vi "Server_v2.vi"() -> ()   [LabVIEW 2016]
uses:
  <vilib>/rvi/eio/common/nirviEmuClasses.ctl
  <vilib>/rvi/Emulation/niFpgaSctlEmulationGetInTimedLoop.vi
  <vilib>/rvi/Emulation/niFpgaProcessEmulError.vi
  <vilib>/rvi/eio/common/nirviEmuTemplateMethod_errors.vi
  <vilib>/rvi/Emulation/niFpgaEmulationIsFPGAContextNoSignature.vi
  <vilib>/rvi/DataTransferAndStorage/Container/Common/niFpgaContainerGetUniqueNameForEmu.vi
  <vilib>/rvi/Memory/Memory_Emulation/niFpgaMemoryEmulationCacheClearOnFirstRun.vi
  <vilib>/rvi/Memory/Memory_Emulation/nirvimemoryEmulationManagerCache_MakeExclusive.vi
  <vilib>/rvi/Memory/Memory_Emulation/niFpgaMemoryEmulationValidateCache.vi
  <vilib>/rvi/Memory/Memory_Emulation/nirvimemoryEmulationManagerCache_InsertValue.vi
  <vilib>/Utility/error.llb/Clear Errors.vi
  <vilib>/rvi/Memory/Memory_Emulation/nirvimemoryEmulationManagerCache_ReleaseExclusive.vi
  <vilib>/rvi/Memory/Memory_Emulation/nirvimemoryEmulationManagerCache_GetValue.vi
  <vilib>/rvi/Memory/Memory_Emulation/nirvimemoryEmulationManagerCache_SetValue.vi
  <vilib>/rvi/Emulation/niFpgaGetClockAttributes.vi
  <vilib>/rvi/Emulation/niFpgaEmulationReportErrorSimple.vi
  <vilib>/rvi/Emulation/niFpgaCriticalErrorInLSC.vi
  <vilib>/rvi/eio/common/nirviEmuTemplateMethod_noerrors.vi
  <vilib>/rvi/errors/niFpgaSetErrorForExecOnDevCompSimple.vi
  <vilib>/rvi/eio/common/nirviEmuReportErrorAndStop.vi
  <vilib>/rvi/FIFO/Fifo_Resource/nirvififoEmulationSetSize.vi
  <vilib>/rvi/FIFO/Fifo_Resource/nirviFifoEmulationQueueMgr.vi
  <instcachedir>/0/nirviFifoEmulationQueueMgr_E5CAEC123FF24DC58D834DCA3CDAA9B5.lvgen/nirviFifoEmulationQueueMgr_E5CAEC123FF24DC58D834DCA3CDAA9B5_001.vi
  <vilib>/rvi/FIFO/Fifo_Resource/nirvififoEmulationCreateLock.vi
  <vilib>/rvi/FIFO/Fifo_Resource/nirvififoEmulationObtainLock.vi
  <vilib>/rvi/FIFO/Fifo_Resource/nirvififoEmulationReleaseLock.vi
  <vilib>/rvi/occurrence/nirviWaitOnOccurrenceBase.vi
  <vilib>/rvi/errors/nirviReportUnexpectedCaseInternalError.vi
  <vilib>/rvi/errors/nirviReportUnexpectedCaseInternalError (U32).vi
  <vilib>/rvi/FIFO/Fifo_Resource/nirvififoEmulationDetermineInputValidOut.vi
  <vilib>/eio/EIOGrowableMethodNode/genericMethod/EIOGrowableMethodNode.xnode
  <vilib>/rvi/eio/nirviEIOMethodImplementation/nirviEIOMethodImplementation.xnode
  <vilib>/rvi/eio/nirviErrorMerge/nirviErrorMerge.xnode
  <vilib>/rvi/DataTransferAndStorage/Container/XNode/niFpgaContainer.xnode
  <vilib>/rvi/DataTransferAndStorage/Register/Emulation/niFpgaRegisterEmulation.vi
  <vilib>/eio/EIONode/EIONode.xnode
  <vilib>/rvi/FIFO/Fifo_Resource/nirvififoEmulationRead.vi
  <vilib>/rvi/FIFO/Fifo_Resource/nirvififoEmulationWrite.vi
panel:
  out "Temperatures":T1
  in  "Spare DC Relay 1":bool
  in  "AC Spare":bool
  in  "Spare DC Relay 2":bool
  out "Sensor Status":u8
  in  "PAS Laser 1 Enable":bool
  in  "PAS Laser 2 Enable":bool
  in  "CRD Laser Enable":bool
  in  "Fan Voltage":i16
  in  "CRD Heater Enable":bool
  in  "PAS Heater 2":bool
  in  "PAS Heater 1":bool
  in  "pas_frequency":u64
  in  "Vacuum Pump":bool
  in  "Error Mode":bool
  in  "PAS Speaker Enable":bool
  in  "O2 Add":bool
  in  "uv light enable":bool
  in  "Fan Enable":bool
  in  "O3 Add":bool
  in  "Filter Ctl":bool
  in  "Transmit?":bool
  in  "CRDSampData":u32
  in  "Speaker":cluster{"Vscale":fxp<+,32,0>, "Offset":i16}
  in  "Stop":bool
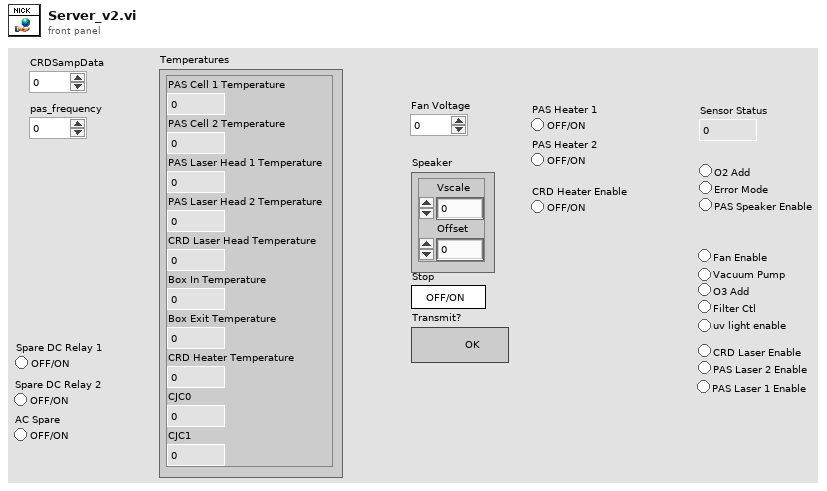
[diagram p1: front panel]
types:
  T1 = cluster{"PAS Cell 1 Temperature":fxp<+/-,24,-2>, "PAS Cell 2 Temperature":fxp<+/-,24,-2>, "PAS Laser Head 1 Temperature":fxp<+/-,24,-2>, "PAS Laser Head 2 Temperature":fxp<+/-,24,-2>, "CRD Laser Head Temperature":fxp<+/-,24,-2>, "Box In Temperature":fxp<+/-,24,-2>, "Box Exit Temperature":fxp<+/-,24,-2>, "CRD Heater Temperature":fxp<+/-,24,-2>, "CJC0":fxp<+/-,24,-2>, "CJC1":fxp<+/-,24,-2>}
  T2 = typedef "nirviEmuClasses.ctl" = enum16{"IO Read", "IO Write", "Method", "Property Read", "Property Write"}
  T3 = cluster{"PAS Cell 1 Temperature":fxp<+/-,24,-2>, "PAS Cell 2 Temperature":fxp<+/-,24,-2>, "PAS Laser Head 1 Temperature":fxp<+/-,24,-2>, "PAS Laser Head 2 Temperature":fxp<+/-,24,-2>, "CRD Laser Head Temperature":fxp<+/-,24,-2>, "Box In Temperature":fxp<+/-,24,-2>, "Box Exit Temperature":fxp<+/-,24,-2>, "CRD Heater Temperature":fxp<+/-,24,-2>, "Mod5/CJC0":fxp<+/-,24,-2>, "Mod5/CJC1":fxp<+/-,24,-2>}
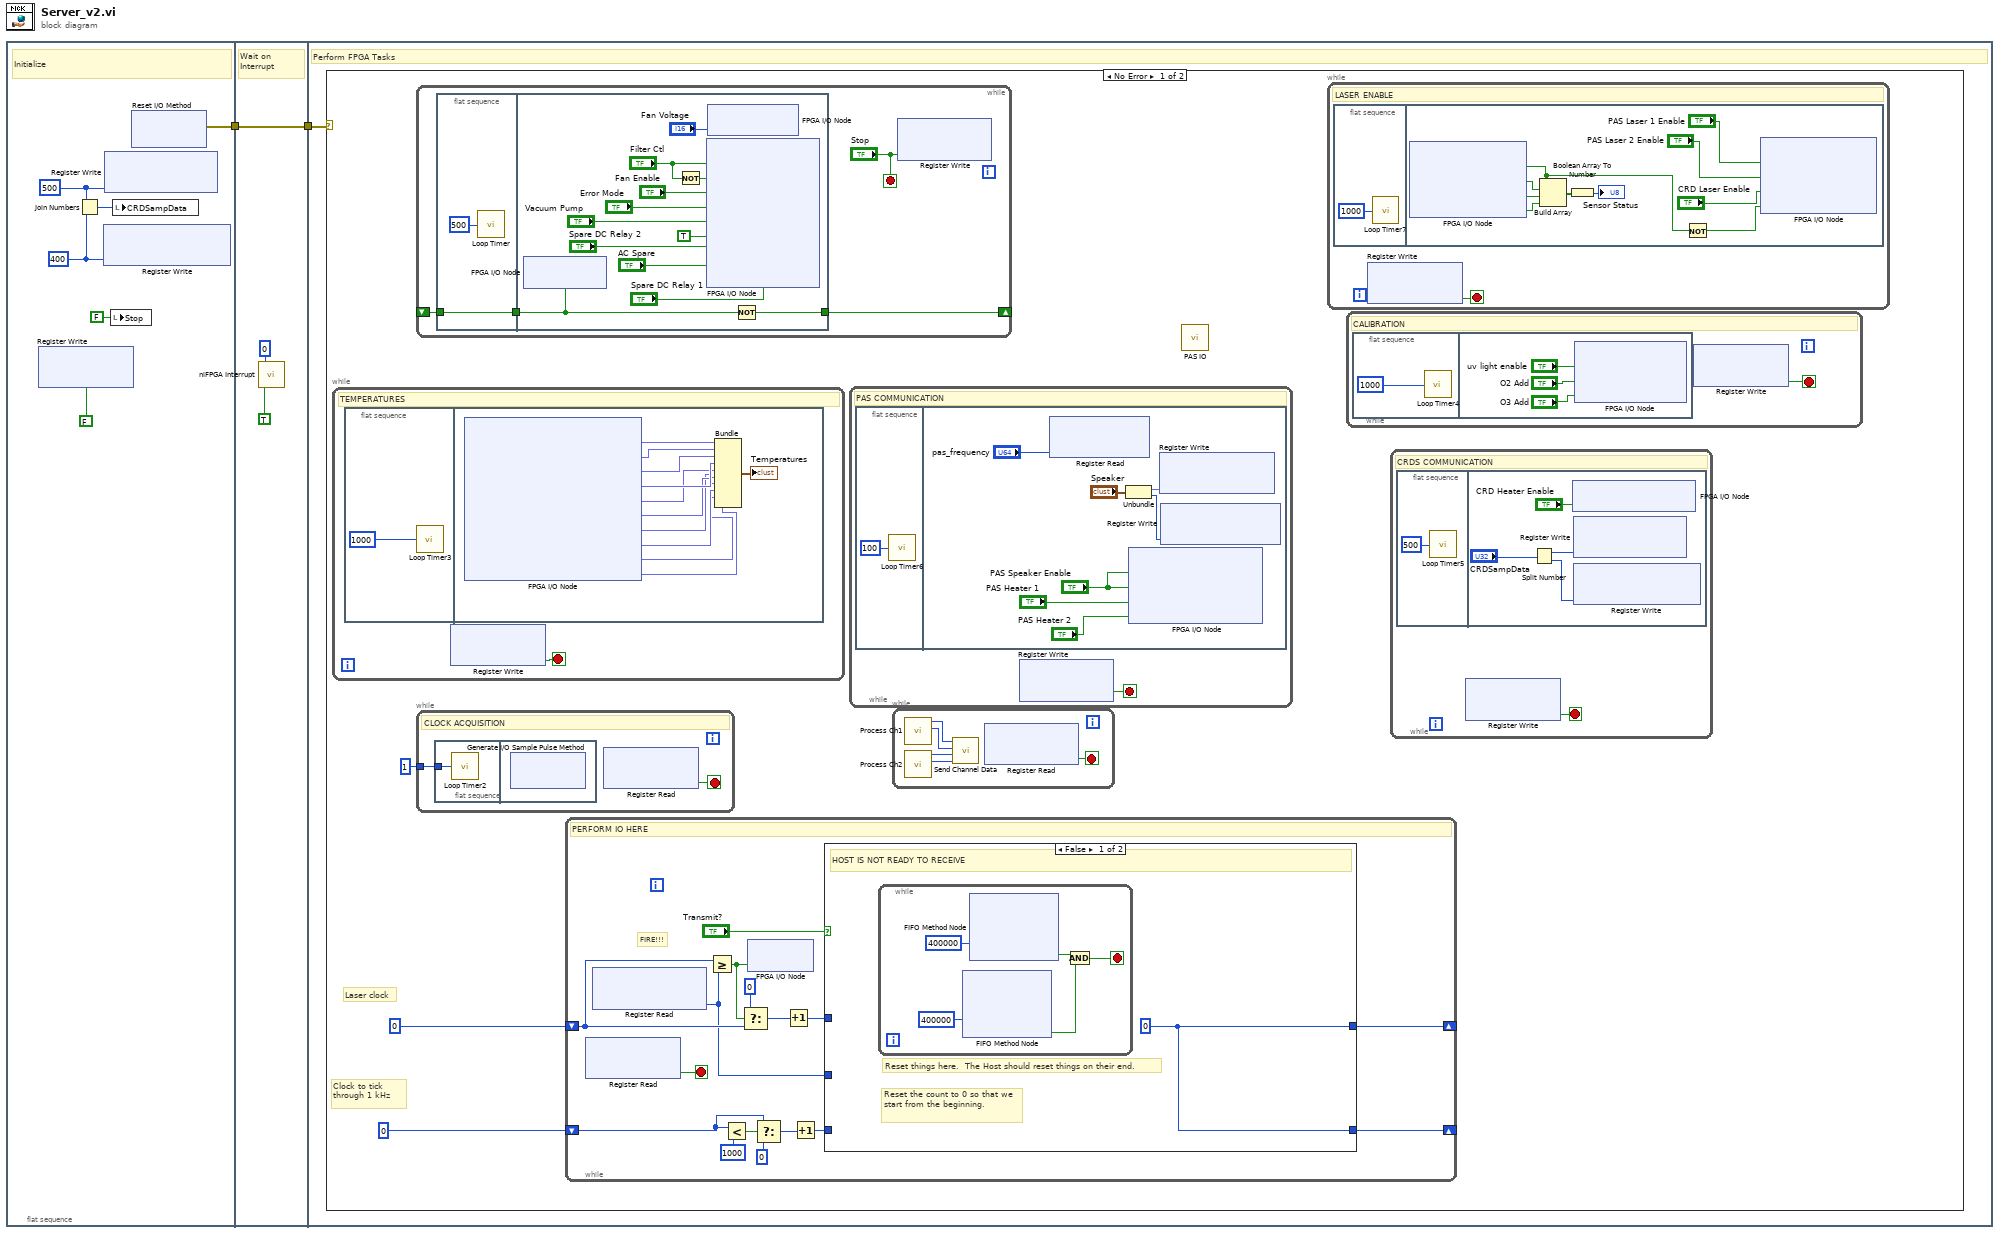
[diagram p0: block diagram]
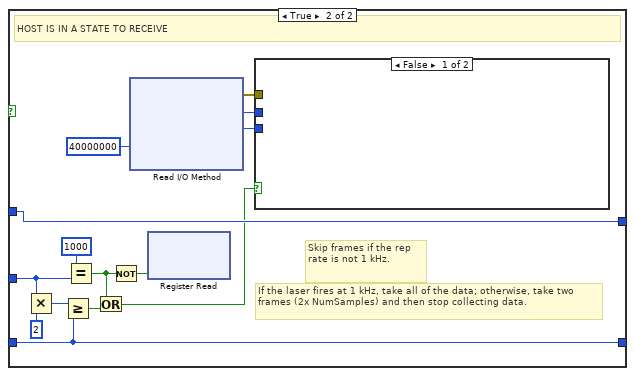
[diagram p2: hidden frame]
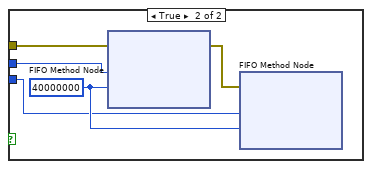
[diagram p3: hidden frame]
diagram:
  n1 = flat-sequence {
    tunnel: [w8] -> w2
    tunnel: w2 -> [w55]
    tunnel: [w55] -> w1
    tunnel: w1 -> [w56]
    frame #0 {
      w5 = u16 500 ("Data")
      w4 = u16 400 ("Data")
      # "Initialize"
      n2 = xnode ("Register Write")("Data"=FALSE) -> ()  [unwired: 1 in, 1 out]
      n3 = Join Numbers(hi=w5, lo=w4) -> ((hi.lo)=w3:u32)
      n4 = xnode ("Register Write")("Data"=w4) -> ()  [unwired: 1 in, 1 out]
      n5 = xnode ("Register Write")("Data"=w5) -> ()  [unwired: 1 in, 1 out]
      n6 = local write "Stop"(FALSE ("Stop")) -> ()
      n7 = local write "CRDSampData"(w3) -> ()
      n8 = xnode "Reset I/O Method"() -> ("error out"=w8:errorcluster)  [unwired: 2 in, 1 out]
    }
    frame #1 {
      # "Wait on Interrupt"
      n9 = call <vilib>:"niFPGA Interrupt.vi"("Wait Until Cleared (F)"=TRUE ("Wait Until Cleared"), "IRQ Number (0)"=u8 0 ("IRQ Number")) -> ()  [unwired: 1 in]
    }
    frame #2 {
      # "Perform FPGA Tasks"
      n10 = case shown="No Error" w56 {
        frame No Error {
          # "Laser clock"
          # "Clock to tick through 1 kHz"
          n11 = while {
            stop <- w255 stop-if-true
            # "TEMPERATURES"
            n12 = flat-sequence {
              frame #0 {
                n13 = call "Loop Timer3"("Count(mSec)"=u32 1000 ("Sample Period (uSec)")) -> ()  [unwired: 1 out]
              }
              frame #1 {
                n14 = xnode "FPGA I/O Node"() -> ("PAS Cell 1 Temperature"=w267:fxp<+/-,24,-2>, "PAS Cell 2 Temperature"=w266:fxp<+/-,24,-2>, "PAS Laser Head 1 Temperature"=w265:fxp<+/-,24,-2>, "PAS Laser Head 2 Temperature"=w264:fxp<+/-,24,-2>, "CRD Laser Head Temperature"=w263:fxp<+/-,24,-2>, "Box In Temperature"=w262:fxp<+/-,24,-2>, "Box Exit Temperature"=w261:fxp<+/-,24,-2>, "CRD Heater Temperature"=w260:fxp<+/-,24,-2>, "Mod5/CJC0"=w259:fxp<+/-,24,-2>, "Mod5/CJC1"=w258:fxp<+/-,24,-2>)  [unwired: 10 in, 10 out]
                n15 = Bundle("PAS Cell 1 Temperature"=w267, "PAS Cell 2 Temperature"=w266, "PAS Laser Head 1 Temperature"=w265, "PAS Laser Head 2 Temperature"=w264, "CRD Laser Head Temperature"=w263, "Box In Temperature"=w262, "Box Exit Temperature"=w261, "CRD Heater Temperature"=w260, "Mod5/CJC0"=w259, "Mod5/CJC1"=w258) -> (→"Temperatures":T3)  [unwired: 1 in]
              }
            }
            n16 = xnode ("Register Write")() -> ("Data"=w255:bool)  [unwired: 1 in, 1 out]
          }
          n17 = while {
            shift-right: [w271] -> _
            shift-left: _ -> [w270]
            stop <- "Stop" stop-if-true
            n18 = flat-sequence {
              tunnel: w270 -> [w273]
              tunnel: [w273] -> w268
              tunnel: [w285] -> w271
              tunnel: w268 -> [w284]
              frame #0 {
                n19 = call "Loop Timer"("Count(mSec)"=u32 500) -> ()  [unwired: 1 out]
              }
              frame #1 {
                n20 = xnode "FPGA I/O Node"("Heartbeat"=w284) -> ()  [unwired: 1 in, 1 out]
                n21 = Not(x="Filter Ctl") -> (.not. x?=w282:bool)
                n22 = xnode "FPGA I/O Node"("hb 1 ctl 1"="Filter Ctl", "hb 1 ctl 2"=w282, "Fan Enable"="Fan Enable", "Error Mode"="Error Mode", "Vacuum Pump"="Vacuum Pump", "USB Hub Relay"=TRUE, "Spare DC Relay 2"="Spare DC Relay 2", "AC Spare"="AC Spare", "Spare DC Relay 1"="Spare DC Relay 1") -> ()  [unwired: 9 in, 9 out]
                n23 = xnode "FPGA I/O Node"("Fan Voltage"="Fan Voltage") -> ()  [unwired: 1 in, 1 out]
                n24 = Not(x=w284) -> (.not. x?=w285:bool)
              }
            }
            n25 = xnode ("Register Write")("Data"="Stop") -> ()  [unwired: 1 in, 1 out]
          }
          n26 = while {
            tunnel: u32 1 ("Sample Period (uSec)") -> [w227]
            stop <- w226 stop-if-true
            # "CLOCK ACQUISITION"
            n27 = flat-sequence {
              tunnel: w227 -> [w228]
              frame #0 {
                n28 = call "Loop Timer2"("Count(uSec)"=w228) -> ()  [unwired: 1 out]
              }
              frame #1 {
                n29 = xnode "Generate I/O Sample Pulse Method"() -> ()  [unwired: 2 in, 2 out]
              }
            }
            n30 = xnode ("Register Read")() -> ("Data"=w226:bool)  [unwired: 1 in, 1 out]
          }
          n31 = while {
            shift-right: [w89] -> _
            shift-left: u16 0 ("Number of Samples") -> [w90]
            shift-right: [w81] -> _
            shift-left: u16 0 ("Number of Samples") -> [w79]
            stop <- w78 stop-if-true
            # "FIRE!!!"
            # "PERFORM IO HERE"
            n32 = xnode ("Register Read")() -> ("Data"=w78:bool)  [unwired: 1 in, 1 out]
            n33 = xnode ("Register Read")() -> ("Data"=w84:u16)  [unwired: 1 in, 1 out]
            n34 = Greater Or Equal?(x=w90, y=w84) -> (x >= y?=w91:bool)
            n35 = Less?(x=w79, y=u16 1000) -> (x < y?=w83:bool)
            n36 = Select(t=u16 0 ("Number of Samples"), s=w91, f=w90) -> (s? t:f=w88:u16)
            n37 = xnode "FPGA I/O Node"("CRDS"=w91) -> ()  [unwired: 1 in, 1 out]
            n38 = Select(t=w79, s=w83, f=u16 0 ("Number of Samples")) -> (s? t:f=w86:u16)
            n39 = Increment(x=w88) -> (x+1=w87:u16)
            n40 = Increment(x=w86) -> (x+1=w82:u16)
            n41 = case shown="False" "Transmit?" {
              tunnel: w87 -> [_ w112]
              tunnel: [w93 w112] -> w89
              tunnel: w84 -> [_ w108]
              tunnel: w82 -> [_ w103]
              tunnel: [w93 w103] -> w81
              frame False {
                w93 = u16 0 ("Number of Samples")
                # "Reset things here.  The Host should reset things on their end."
                # "Reset the count to 0 so that we start from the beginning."
                # "HOST IS NOT READY TO RECEIVE"
                n42 = while {
                  stop <- w94 stop-if-true
                  n43 = xnode ("FIFO Method Node")("Timeout"=400000) -> ("Timed Out?"=w95:bool)  [unwired: 1 in, 2 out]
                  n44 = xnode ("FIFO Method Node")("Timeout"=400000) -> ("Timed Out?"=w96:bool)  [unwired: 1 in, 2 out]
                  n45 = And(x=w96, y=w95) -> (x .and. y?=w94:bool)
                }
              }
              frame True {
                # "Skip frames if the rep rate is not 1 kHz."
                # "If the laser fires at 1 kHz, take all of the data; otherwise, take two frames (2x NumSamples) and then stop collecting data."
                # "HOST IS IN A STATE TO RECEIVE"
                n46 = Multiply(x=w108, y=u16 2) -> (x*y=w106:u16)
                n47 = Greater Or Equal?(x=w106, y=w103) -> (x >= y?=w105:bool)
                n48 = Equal?(x=u16 1000, y=w108) -> (x = y?=w110:bool)
                n49 = Or(x=w110, y=w105) -> (x .or. y?=w104:bool)
                n50 = Not(x=w110) -> (.not. x?=w109:bool)
                n51 = xnode "Read I/O Method"("Timeout"=40000000) -> ("error out"=w100:errorcluster, "CRD Las Ch 1"=w101:i16, "CRD Las Ch 2"=w99:i16)  [unwired: 3 in, 3 out]
                n52 = xnode ("Register Read")("Data"=w109) -> ()  [unwired: 1 in, 1 out]
                n53 = case shown="False" w104 {
                  tunnel: w101 -> [_ w225]
                  tunnel: w100 -> [_ w224]
                  tunnel: w99 -> [_ w222]
                  frame False {
                  }
                  frame True {
                    w223 = 40000000 ("Timeout")
                    n54 = xnode ("FIFO Method Node")("Element"=w225, "Timeout"=w223, "error in (no error)"=w224) -> ("error out"=w221:errorcluster)  [unwired: 1 in, 2 out]
                    n55 = xnode ("FIFO Method Node")("Element"=w222, "Timeout"=w223, "error in (no error)"=w221) -> ()  [unwired: 1 in, 3 out]
                  }
                }
              }
            }
          }
          n56 = while {
            stop <- w235 stop-if-true
            # "PAS COMMUNICATION"
            n57 = flat-sequence {
              frame #0 {
                n58 = call "Loop Timer6"("Count(mSec)"=u32 100) -> ()  [unwired: 1 out]
              }
              frame #1 {
                n59 = xnode ("Register Read")("Data"="pas_frequency") -> ()  [unwired: 1 in, 1 out]
                n60 = Unbundle("Speaker") -> ("Vscale"=w243:fxp<+,32,0>, "Offset"=w242:i16)
                n61 = xnode "FPGA I/O Node"("PAS Speaker Enable 1"="PAS Speaker Enable", "PAS Speaker Enable 2"="PAS Speaker Enable", "PAS Heater 1"="PAS Heater 1", "PAS Heater 2"="PAS Heater 2") -> ()  [unwired: 4 in, 4 out]
                n62 = xnode ("Register Write")("Data"=w243) -> ()  [unwired: 1 in, 1 out]
                n63 = xnode ("Register Write")("Data"=w242) -> ()  [unwired: 1 in, 1 out]
              }
            }
            n64 = xnode ("Register Write")() -> ("Data"=w235:bool)  [unwired: 1 in, 1 out]
          }
          n65 = while {
            stop <- w76 stop-if-true
            n66 = call "Process Ch1.vi"() -> ("Max1"=w74:u32, "Max0"=w75:u32)  [unwired: 10 in]
            n67 = call "Process Ch2.vi"() -> ("Max4"=w72:u32, "Max3"=w73:u32)  [unwired: 10 in]
            n68 = call "Send Channel Data.vi"("Max3"=w72, "Max2"=w73, "Max1"=w74, "Max0"=w75) -> ()  [unwired: 7 in, 1 out]
            n69 = xnode ("Register Read")() -> ("Data"=w76:bool)  [unwired: 1 in, 1 out]
          }
          n70 = call "PAS IO.vi"() -> ()  [unwired: 20 in]
          n71 = while {
            stop <- w60 stop-if-true
            # "LASER ENABLE"
            n72 = flat-sequence {
              frame #0 {
                n73 = call "Loop Timer7"("Count(mSec)"=u32 1000) -> ()  [unwired: 1 out]
              }
              frame #1 {
                n74 = xnode "FPGA I/O Node"() -> ("Interlock Sense"=w63:bool, "hb 1 status 1"=w67:bool, "hb 1 status 2"=w66:bool, "Soft Power Down"=w65:bool)  [unwired: 4 in, 4 out]
                n75 = Build Array(w63, w67, w66, w65) -> (w64:bool[])
                n76 = Boolean Array To Number(Boolean array=w64) -> (number=→"Sensor Status":u8)
                n77 = Not(x=w63) -> (.not. x?=w62:bool)
                n78 = xnode "FPGA I/O Node"("PAS Laser Relay 1"="PAS Laser 1 Enable", "PAS Laser Relay 2"="PAS Laser 2 Enable", "CRD Laser Enable"="CRD Laser Enable", "Interlock Sense"=w62) -> ()  [unwired: 4 in, 4 out]
              }
            }
            n79 = xnode ("Register Write")() -> ("Data"=w60:bool)  [unwired: 1 in, 1 out]
          }
          n80 = while {
            stop <- w250 stop-if-true
            # "CALIBRATION"
            n81 = flat-sequence {
              frame #0 {
                n82 = call "Loop Timer4"("Count(mSec)"=u32 1000 ("Sample Period (uSec)")) -> ()  [unwired: 1 out]
              }
              frame #1 {
                n83 = xnode "FPGA I/O Node"("uv light enable"="uv light enable", "Solenoid Relay 1"="O2 Add", "Solenoid Relay 2"="O3 Add") -> ()  [unwired: 3 in, 3 out]
              }
            }
            n84 = xnode ("Register Write")() -> ("Data"=w250:bool)  [unwired: 1 in, 1 out]
          }
          n85 = while {
            stop <- w244 stop-if-true
            # "CRDS COMMUNICATION"
            n86 = flat-sequence {
              frame #0 {
                n87 = call "Loop Timer5"("Count(mSec)"=u32 500) -> ()  [unwired: 1 out]
              }
              frame #1 {
                n88 = Split Number(x="CRDSampData") -> (hi(x)=w248:u16, lo(x)=w249:u16)
                n89 = xnode "FPGA I/O Node"("CRD Heater Enable"="CRD Heater Enable") -> ()  [unwired: 1 in, 1 out]
                n90 = xnode ("Register Write")("Data"=w248) -> ()  [unwired: 1 in, 1 out]
                n91 = xnode ("Register Write")("Data"=w249) -> ()  [unwired: 1 in, 1 out]
              }
            }
            n92 = xnode ("Register Write")() -> ("Data"=w244:bool)  [unwired: 1 in, 1 out]
          }
        }
        frame Error {
        }
      }
    }
  }
